vi "Wait-for-assert-safe.vi"(8 "error in (no error)":errorcluster, 11 "Object ref in":T1) -> (0 "error out":errorcluster, 3 "Object ref out":T1)   [LabVIEW 2013, in "PowderDeposition.lvlib" / "PD-Main.lvclass"]
uses:
  PD-Main.lvclass
  Object-reference.ctl
  PD-Main.lvclass/PD-Main.ctl
  Motor/Motor.lvclass
  Custom-errors.ctl
  Read Motor assembly.vi
  Assembly/Motor-assembly.lvclass
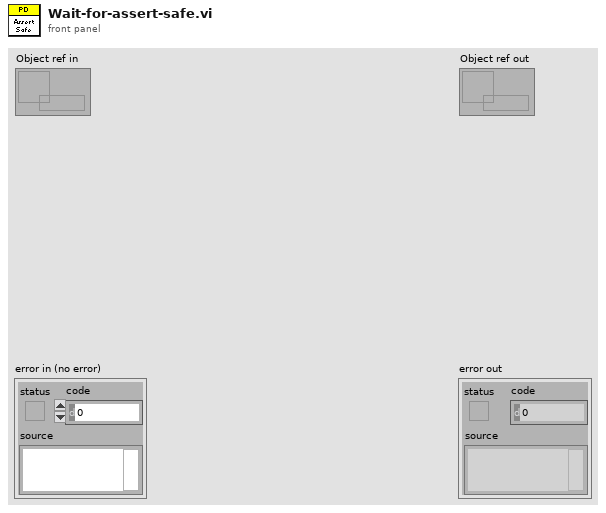
[diagram p1: front panel]
types:
  T1 = typedef "PowderDeposition.lvlib/PD-Main.lvclass/Object-reference.ctl" = refnum<data-value>
  T2 = typedef "PowderDeposition.lvlib/PD-Main.lvclass/Custom-errors.ctl" = enum16{"Not implemented", "Command not recognized", "Invalid input", "Timeout", "Load file failed", "Action failed", "Action invalid", "Motor inactive", "Not in range", "Unsafe state"}
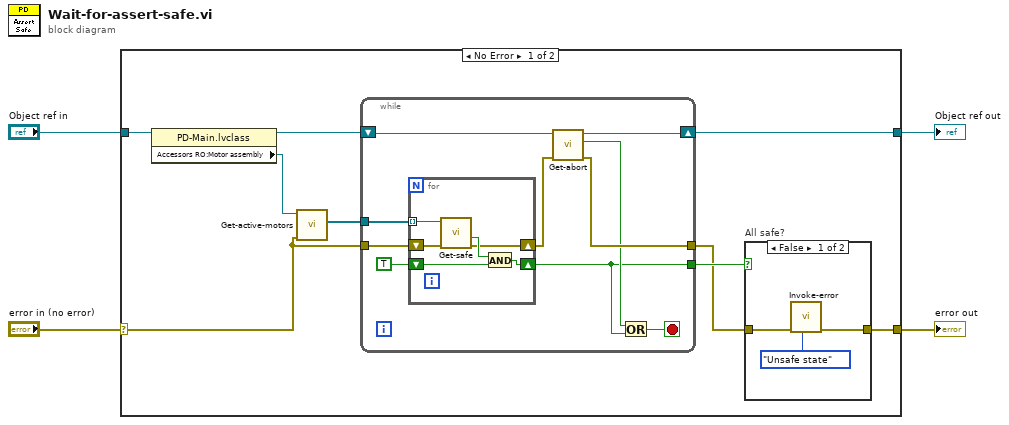
[diagram p0: block diagram]
diagram:
  n1 = case shown="No Error" "error in (no error)" {
    selector: "error in (no error)" -> [w9 w35]
    tunnel: [w12 w35] -> w3
    tunnel: [w5 w34] -> w1
    tunnel: "Object ref in" -> [w13 w34]
    frame No Error {
      n2 = property class="PD-Main.lvclass"(reference=w13) -> (reference out=w8:T1, "Accessors RO:Motor assembly"=w11:refnum<class "Motor-assembly.lvclass">)  [unwired: 1 in, 1 out]
      n3 = call "Get-active-motors.vi"("error in (no error)"=w9, "Available motors in"=w11) -> ("Active motors"=w10:refnum<class "Motor.lvclass">[])  [unwired: 7 in, 2 out]
      n4 = while {
        tunnel: w10 -> [w27]
        tunnel: w9 -> [w25]
        shift-right: [w23] -> w5
        shift-left: w8 -> [w24]
        tunnel: [w21] -> w6
        tunnel: [w18] -> w7
        stop <- w20 stop-if-true
        n5 = for {
          tunnel: w27 -> [w33] mode=indexing
          shift-right: [w31] -> w18
          shift-left: TRUE -> [w30]
          shift-right: [w28] -> w22
          shift-left: w25 -> [w29]
          n6 = call-dynamic "Get-safe.vi"("error in (no error)"=w29, "Motor in"=w33) -> ("error out"=w28:errorcluster, "Safe?"=w32:bool)  [unwired: 7 in, 1 out]
          n7 = And(x=w32, y=w30) -> (x .and. y?=w31:bool)
        }
        n8 = call "Get-abort.vi"("error in (no error)"=w22, "Object ref in"=w24) -> ("error out"=w21:errorcluster, "Abort"=w19:bool, "Object ref out"=w23:T1)  [unwired: 7 in]
        n9 = Or(x=w19, y=w18) -> (x .or. y?=w20:bool)
      }
      n10 = case "All safe?" shown="False" w7 {
        tunnel: [w16 w17] -> w12
        tunnel: w6 -> [w14 w17]
        frame False {
          n11 = call "Invoke-error.vi"("Error"=Custom-errors."Unsafe state", "error in (no error)"=w14) -> ("error out"=w16:errorcluster)  [unwired: 9 in]
        }
        frame True {
        }
      }
    }
    frame Error {
    }
  }
  "error out" <- w3
  "Object ref out" <- w1
